vi "Update Substatus.vi"(8 "error in (no error)":errorcluster, 9 "Status":string, 10 "Name":string, 11 "Module in":refnum<class "Module.lvclass">) -> (0 "error out":errorcluster, 3 "Module out":refnum<class "Module.lvclass">)   [LabVIEW 2020, in "Volatus.lvlib" / "Module.lvclass"]
uses:
  Module.lvclass
  Module.lvclass/Module.ctl
  Module Substatus.ctl
  Volatus.lvlib
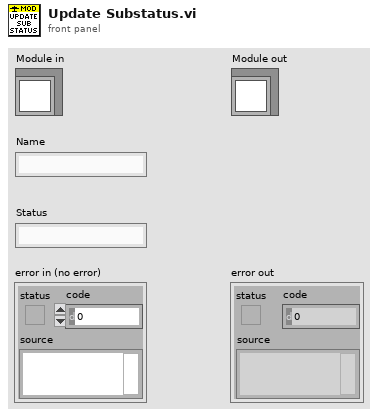
[diagram p1: front panel]
types:
  T1 = typedef "Volatus.lvlib/Module Substatus.ctl" = cluster{"Hierarchy":string[], "Name":string, "Status":string}
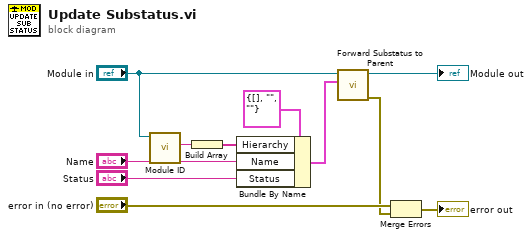
[diagram p0: block diagram]
diagram:
  n1 = call-dynamic "Module ID.vi"("Module in"="Module in") -> ("Module ID"=w10:string)  [unwired: 10 in]
  n2 = Build Array(w10) -> (w7:string[])
  n3 = Bundle By Name(cluster=T1 {"Hierarchy"=[], "Name"="", "Status"=""} ("Module Substatus"), "Hierarchy"=w7, "Name"="Name", "Status"="Status") -> (w3:T1)
  n4 = call "Forward Substatus to Parent.vi"("Module Substatus"=w3, "Module in"="Module in") -> ("error out"=w1:errorcluster, "Module out"=→"Module out":refnum<class "Module.lvclass">)  [unwired: 8 in]
  n5 = Merge Errors("error in (no error)", w1) -> (→"error out":errorcluster)
